vi "Get Number.vi"(8 "error in (no error)":errorcluster, 11 "Number in":refnum<class "Number.lvclass">) -> (0 "error out":errorcluster, 2 "Number":i32, 3 "Number out":refnum<class "Number.lvclass">)   [LabVIEW 2020, in "Number.lvclass"]
uses:
  Number.lvclass
  Number.lvclass/Number.ctl
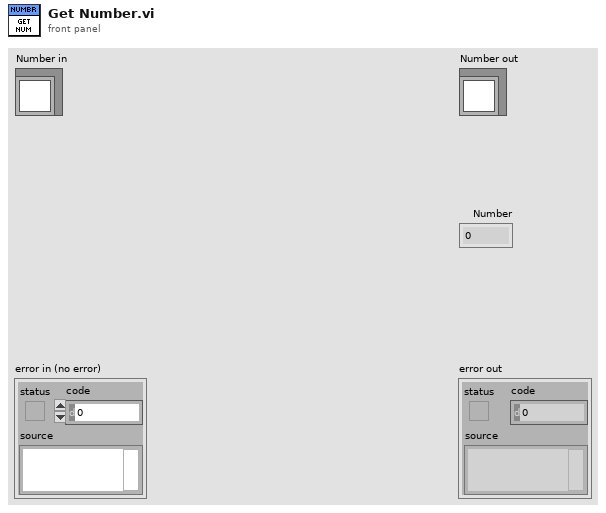
[diagram p1: front panel]
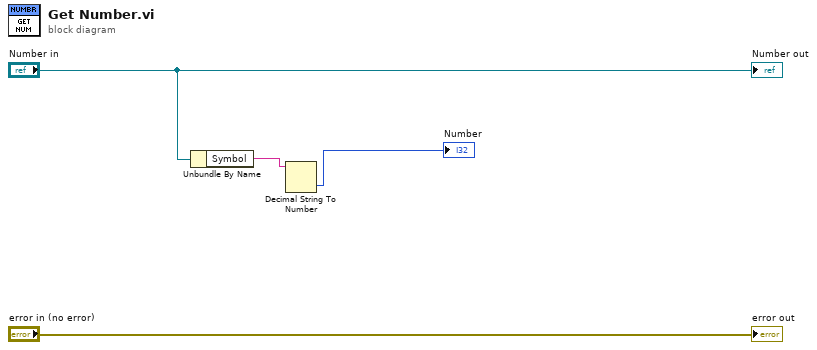
[diagram p0: block diagram]
diagram:
  n1 = Unbundle By Name("Number in") -> ("Symbol"=w2:string)
  n2 = Decimal String To Number(string=w2) -> (number=→"Number":i32)  [unwired: 2 in, 1 out]
  "error out" <- "error in (no error)"
  "Number out" <- "Number in"
